vi "DB_MeasNames.vi"(6 "DB":T1 items=["Server", "Local DB"], 7 "Lista pomiarów":refnum<vi>, 8 "error in":errorcluster, 9 "FilesPath":refnum<vi>, 10 "Lista_Archive":refnum<vi>, 11 "DB in":T2) -> (0 "error out":errorcluster, 3 "DataBase out":T2)   [LabVIEW 2019]
uses:
  <vilib>/addons/database/Connection.llb/Conn ObjectReference.ctl
  TypeDef/#TypeDef_DBMode.ctl
  <vilib>/addons/database/NI_Database_API.lvlib
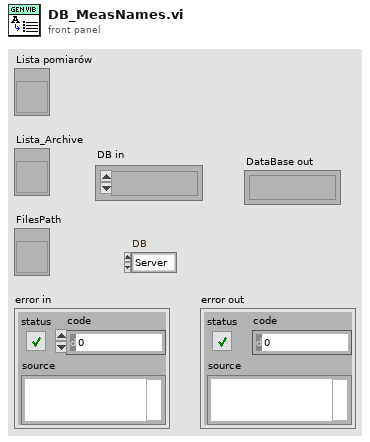
[diagram p1: front panel]
types:
  T1 = typedef "#TypeDef_DBMode.ctl" = u16
  T2 = typedef "NI_Database_API.lvlib/Conn ObjectReference.ctl" = refnum<k1>
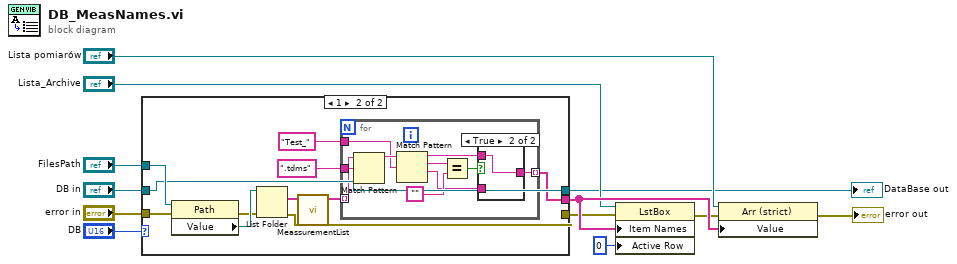
[diagram p0: block diagram]
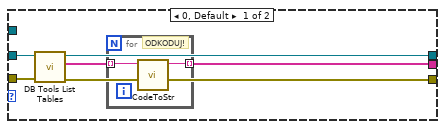
[diagram p2: hidden frame]
diagram:
  n1 = case shown="1" "DB" {
    tunnel: [w13 w21] -> w11
    tunnel: [w17 w25] -> w7
    tunnel: "FilesPath" -> [_ w28]
    tunnel: "error in" -> [w18 w27]
    tunnel: "DB in" -> [w16 w26]
    tunnel: [w15 w26] -> w2
    frame 0, Default {
      n2 = call <vilib>:"DB Tools List Tables.vi"("error in (no error)"=w18, "connection reference"=w16) -> ("error out"=w17:errorcluster, "tables"=w14:string[], "connection reference out"=w15:T2)  [unwired: 3 in]
      n3 = for {
        tunnel: w14 -> [w20] mode=indexing
        tunnel: [w19] -> w13 mode=indexing
        # "ODKODUJ!"
        n4 = call "CodeToStr.vi"("Name in"=w20) -> ("Name out"=w19:string)  [unwired: 10 in]
      }
    }
    frame 1 {
      n5 = property class="Path"(reference=w28, error in=w27) -> (error out=w29:errorcluster, "Value"=w31:path)  [unwired: 1 out]
      n6 = List Folder(path=w31, error in=w29) -> (filenames=w30:string[], error out=w25:errorcluster)  [unwired: 2 in, 2 out]
      n7 = call "MeassurementList.vi"("filenames"=w30) -> ("ListaPomiarów"=w22:string[])  [unwired: 10 in]
      n8 = for {
        tunnel: ".tdms" -> [w41]
        tunnel: "Test_" ("regular expression") -> [w39]
        tunnel: [w33] -> w21 mode=indexing
        tunnel: w22 -> [w32] mode=indexing
        n9 = Match Pattern(string=w32, regular expression=w41) -> (before substring=w40:string)  [unwired: 1 in, 3 out]
        n10 = Match Pattern(string=w40, regular expression=w39) -> (before substring=w35:string, match substring=w38:string, after substring=w34:string)  [unwired: 1 in, 1 out]
        n11 = Equal?(x=w38, y="") -> (x = y?=w36:bool)
        n12 = case shown="True" w36 {
          tunnel: w35 -> [_ w43]
          tunnel: w34 -> [w42 _]
          tunnel: [w42 w43] -> w33
          frame False {
          }
          frame True {
          }
        }
      }
    }
  }
  "DataBase out" <- w2
  n13 = property class="LstBox"(reference="Lista_Archive", error in=w7, "Item Names"=w11, "Active Row"=0 ("Active Row:Active Row Number")) -> (error out=w10:errorcluster)  [unwired: 1 out]
  n14 = property class="Arr (strict)"(reference="Lista pomiarów", error in=w10, "Value"=w11) -> (error out=→"error out":errorcluster)  [unwired: 1 out]
